vi "VI with Splitter.vi"() -> ()   [LabVIEW 2019]
panel:
  in  "String":string
  in  "String 2":string
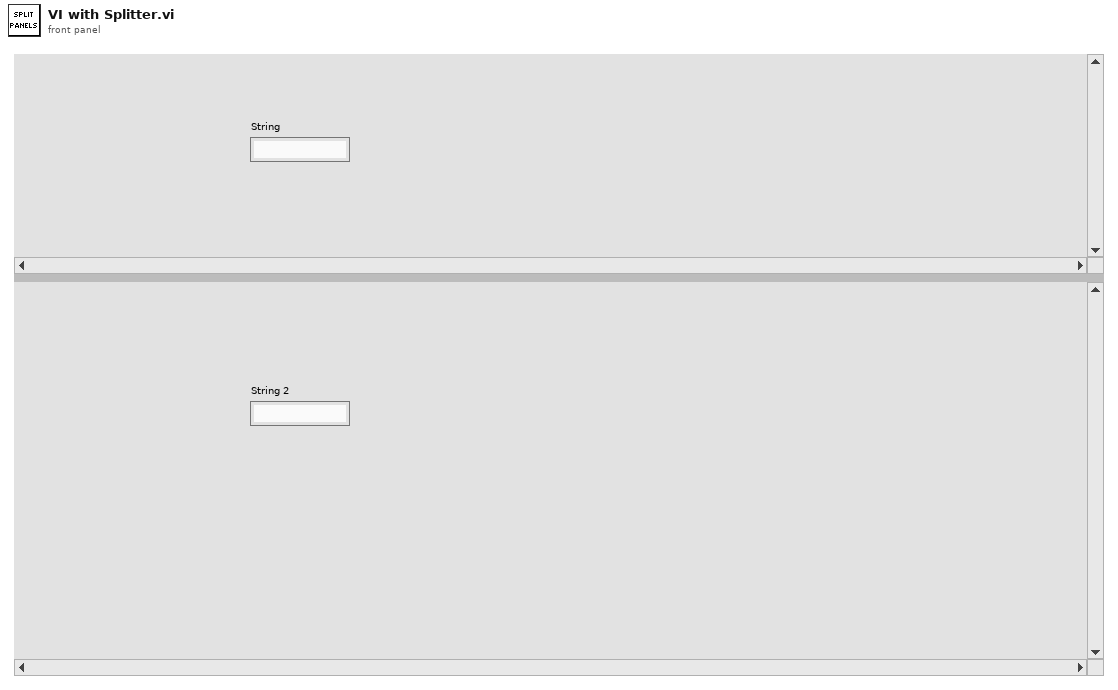
[diagram p1: front panel]
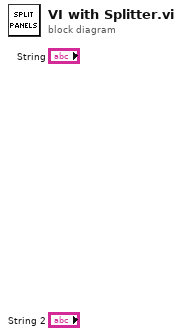
[diagram p0: block diagram]
diagram:
